vi "Launch ConfigurationEditor.vi"(8 "error in (no error)":errorcluster, 11 "Main in":refnum<class "Main.lvclass">) -> (0 "error out":errorcluster, 3 "Main out":refnum<class "Main.lvclass">)   [LabVIEW 2023, in "Main.lvlib" / "Main.lvclass"]
uses:
  Library/Main.lvclass
  builds/Main/ConfigurationEditor.lvlibp/Library/Configuration Editor.lvclass
  Library/Main.lvclass/Main.ctl
  Custom Controls/Components.vi
  builds/Framework/Engine.lvlibp/Managed Actor/Library/Managed Actor.lvclass
  builds/Framework/Engine.lvlibp/Engine/Library/Engine.lvclass
  C:/Users/Public/Documents/Development/builds/Framework/Engine.lvlibp/Engine/Library/Engine.lvclass
  C:/Users/Public/Documents/Development/builds/Framework/Engine.lvlibp/Managed Actor/Library/Managed Actor.lvclass
  builds/Main/Docking.lvlibp/Docking/Docking.lvclass
  C:/Users/Public/Documents/Development/builds/Main/Docking.lvlibp/Docking/Docking.lvclass
  C:/Users/Public/Documents/Development/builds/Framework/Panel Manager.lvlibp/Library/Panel Actor.lvclass
  builds/Framework/Panel Manager.lvlibp/Panel/Panel/Subpanel/Subpanel.lvclass
  C:/Users/Public/Documents/Development/builds/Framework/Panel Manager.lvlibp/Panel/Panel/Panel.lvclass
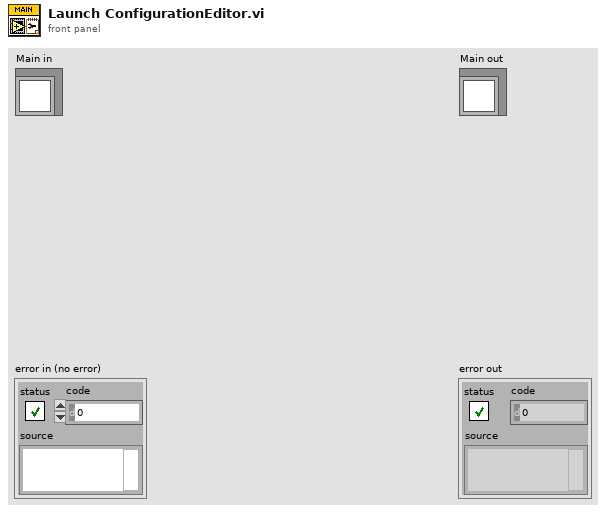
[diagram p1: front panel]
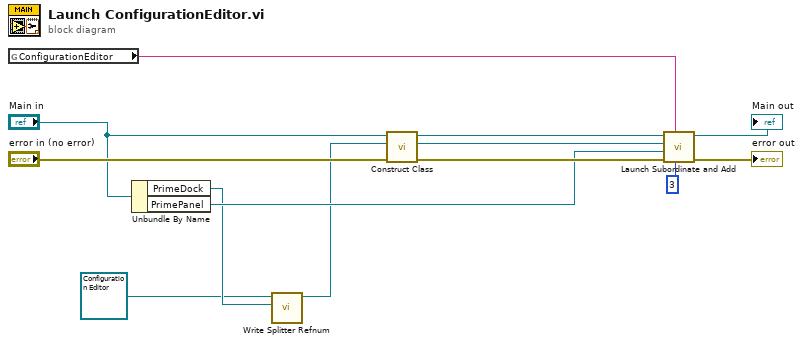
[diagram p0: block diagram]
diagram:
  n1 = global read "Components.vi" "ConfigurationEditor"() -> (w3:string)
  n2 = Unbundle By Name("Main in") -> ("PrimeDock"=w5:refnum<vi>, "PrimePanel"=w7:refnum<class "Subpanel.lvclass">)
  n3 = call "Write Splitter Refnum.vi"("Splitter Refnum"=w5, "Docking in"=refnum<class "Configuration Editor.lvclass"> refnum ("ConfigurationEditor")) -> ("Docking out"=w6:refnum<class "Configuration Editor.lvclass">)  [unwired: 8 in, 1 out]
  n4 = call "Construct Class.vi"("error in (no error)"="error in (no error)", "Actor in"=w6, "Engine in"="Main in") -> ("error out"=w11:errorcluster, "Actor out"=w12:refnum<class "Configuration Editor.lvclass">, "Engine out"=w1:refnum<class "Main.lvclass">)  [unwired: 6 in]
  n5 = call "Launch Subordinate and Add.vi"("PanelIndex"=3, "Identifier"=w3, "error in (no error)"=w11, "Panel"=w7, "Nested Panel Actor"=w12, "Managed Actor in"=w1) -> ("error out"=→"error out":errorcluster, "Managed Actor out"=→"Main out":refnum<class "Main.lvclass">)  [unwired: 4 in]
